vi "Generate Signal.vi"(0 "reference in":refnum<class "Data Generator.lvclass">, 1 "signal type":T1(ring), 2 "frequency":dbl, 3 "amplitude":dbl, 4 "phase":dbl, 5 "Error In":errorcluster) -> (14 "reference out":refnum<class "Data Generator.lvclass">, 15 "Signal Data":T2, 19 "Error Out":errorcluster)   [LabVIEW 2024, in "Data Generator.lvclass"]
doc: "Generates waveform signal according to given parameters."
uses:
  Data Generator.lvclass
  Support/Signal Data.ctl
  <vilib>/measure/NI_MABase.lvlib
panel:
  # "Connector Pane"
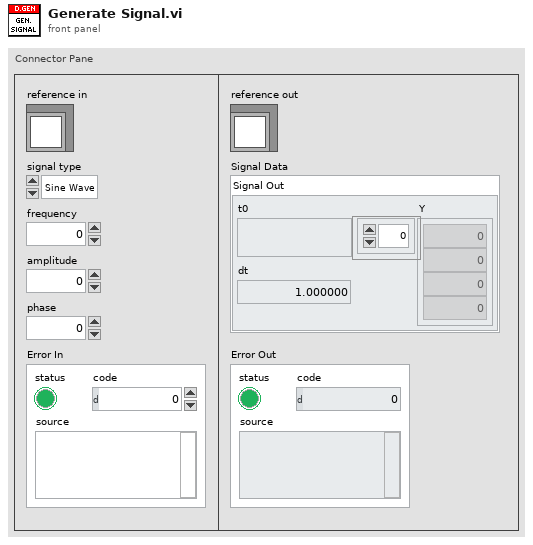
[diagram p1: front panel]
types:
  T1 = enum16{"Sine Wave", "Triangle Wave", "Square Wave", "Sawtooth Wave"}
  T2 = typedef "Signal Data.ctl" = cluster{"Signal Out":waveform(dbl)}
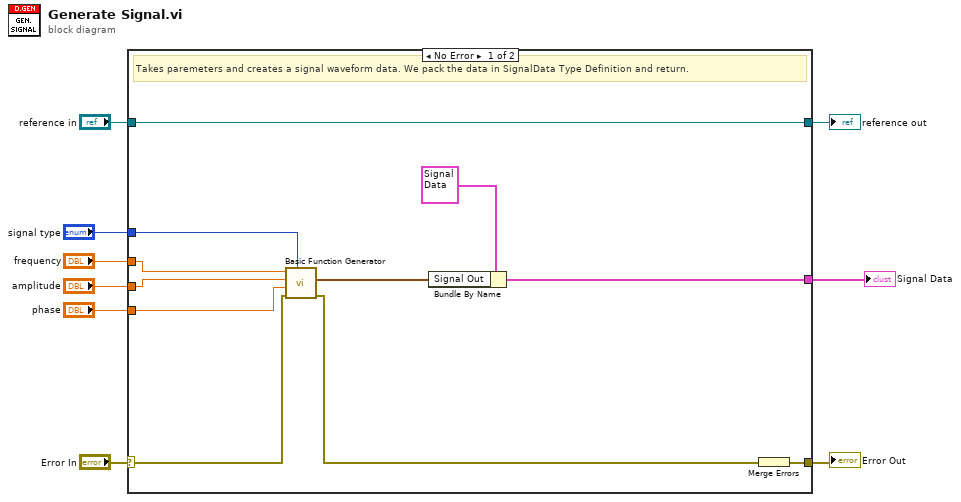
[diagram p0: block diagram]
diagram:
  n1 = case shown="No Error" "Error In" {
    selector: "Error In" -> [w11 w22]
    tunnel: [w19 w22] -> w8
    tunnel: [w20 w21] -> w6
    tunnel: "reference in" -> [w20 w21]
    tunnel: [w18 _] -> w5
    tunnel: "signal type" -> [w15 _]
    tunnel: "frequency" -> [w14 _]
    tunnel: "amplitude" -> [w13 _]
    tunnel: "phase" -> [w12 _]
    frame No Error {
      # "Takes paremeters and creates a signal waveform data. We pack the data in SignalData Type Definition and return."
      n2 = call <vilib>:"Basic Function Generator.vi"("signal type"=w15, "error in (no error)"=w11, "phase"=w12, "amplitude"=w13, "frequency"=w14) -> ("error out"=w10:errorcluster, "signal out"=w16:waveform(dbl))  [unwired: 4 in, 1 out]
      n3 = Bundle By Name(cluster=T2 {"Signal Out"={"t0"=timestamp(0 s since 1904-01-01), "dt"=1.0, "Y"=[]}} ("Data"), "Signal Out"=w16) -> (w18:T2)
      n4 = Merge Errors(w10) -> (w19:errorcluster)
    }
    frame Error {
    }
  }
  "Error Out" <- w8
  "reference out" <- w6
  "Signal Data" <- w5
